vi "InitStacks.vi"(8 "Second":refnum<class "Action.lvclass">[](array[class]), 9 "First":refnum<class "Action.lvclass">[](array[class])) -> (1 "Actions":refnum<class "Action.lvclass">[](array[class]))   [LabVIEW 2025]
uses:
  Action.lvclass
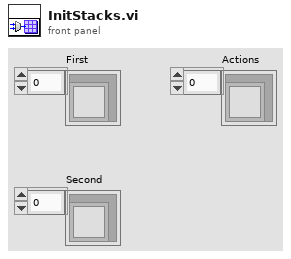
[diagram p1: front panel]
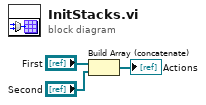
[diagram p0: block diagram]
diagram:
  n1 = Build Array (concatenate)("First", "Second") -> (→"Actions":refnum<class "Action.lvclass">[])
